vi "Write CapturedImage Msg.vi"(10 "Vision.lvlib:CapturedImage Msg.lvclass":refnum<class "CapturedImage Msg.lvclass">, 11 "Vision in":refnum<class "Vision.lvclass">) -> (3 "Vision out":refnum<class "Vision.lvclass">)   [LabVIEW 2021, in "Vision.lvlib" / "Vision.lvclass"]
uses:
  Vision.lvclass
  Vision Messages/CapturedImage Msg/CapturedImage Msg.lvclass
  Vision.lvclass/Vision.ctl
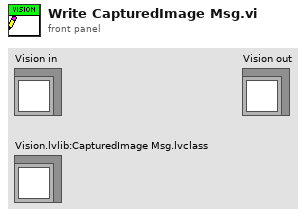
[diagram p1: front panel]
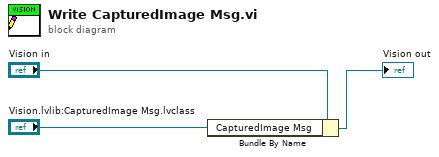
[diagram p0: block diagram]
diagram:
  n1 = Bundle By Name(cluster="Vision in", "CapturedImage Msg"="Vision.lvlib:CapturedImage Msg.lvclass") -> (→"Vision out":refnum<class "Vision.lvclass">)
